vi "VIPMUninstallVIPackagesByName.vi"   [LabVIEW 2016]
uses:
  <vilib>/Wiresmith Technology/G CLI/Argument Parser/Option Class/Option Configuration.ctl
  <vilib>/Wiresmith Technology/G CLI/Argument Parser/Option Class/Argument Type.ctl
  <vilib>/Wiresmith Technology/G CLI/CLI Class/CLI.lvclass
  <vilib>/Wiresmith Technology/G CLI/Argument Parser/Option Set Class/Option Set.lvclass
  <vilib>/Wiresmith Technology/G CLI/Argument Parser/Option Class/Option.lvclass
  <vilib>/JKI/VIPM API/VIPM API_vipm_api.lvlib
types:
  T1 = typedef "Option Parser.lvlib/Option.lvclass/Option Configuration.ctl" = cluster{"Option Type":T2, "Option Labels":string[], "Key":string, "Description":string, "Required":bool, "Default Value":string}
  T2 = typedef "Option Parser.lvlib/Option.lvclass/Argument Type.ctl" = enum16{"flag", "value"}
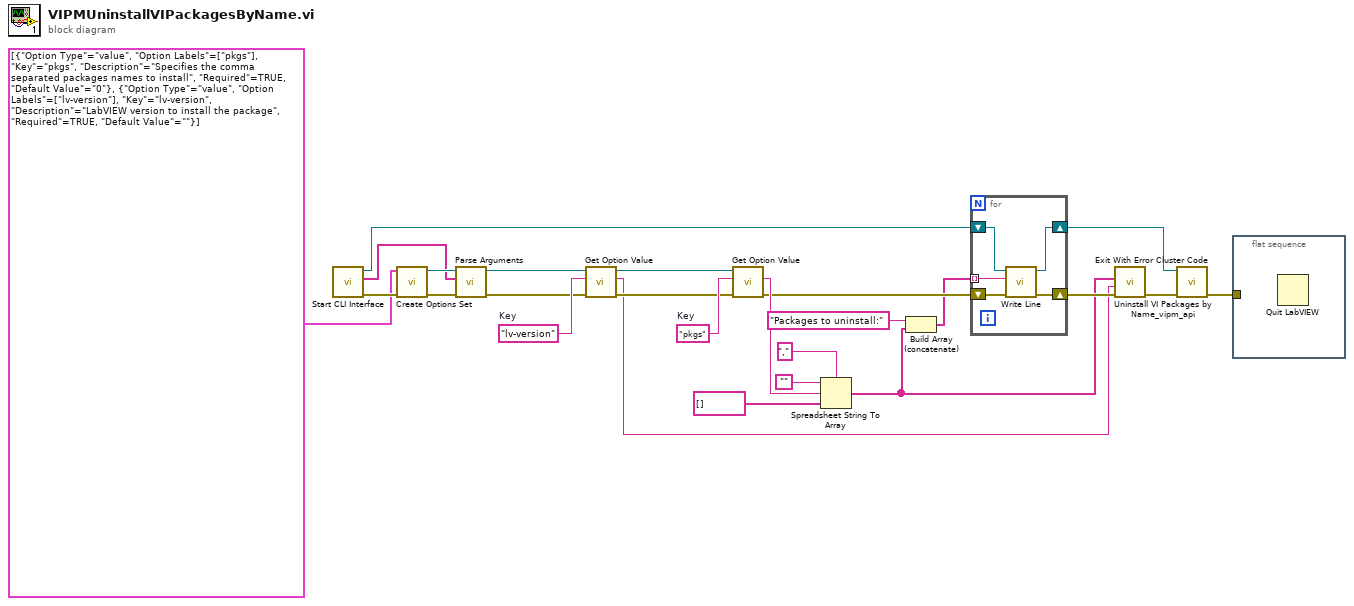
[diagram p0: block diagram]
diagram:
  w12 = "lv-version"  # Key
  w19 = "pkgs"  # Key
  n1 = call <vilib>:"Start CLI Interface.vi"() -> ("error out"=w21:errorcluster, "Custom Parameters"=w22:string[], "CLI out"=w25:refnum<class "CLI.lvclass">)  [unwired: 8 in, 1 out]
  n2 = call <vilib>:"Create Options Set.vi"("error in (no error)"=w21, "Options"=T1[] [{"Option Type"=enum."value", "Option Labels"=["pkgs"], "Key"="pkgs", "Description"="Specifies the comma separated packages names to install", "Required"=TRUE, "Default Value"="0"}, {"Option Type"=enum."value", "Option Labels"=["lv-version"], "Key"="lv-version", "Description"="LabVIEW version to install the package", "Required"=TRUE, "Default Value"=""}]) -> ("error out"=w23:errorcluster, "Option Set out"=w24:refnum<class "Option Set.lvclass">)  [unwired: 8 in]
  n3 = call <vilib>:"Parse Arguments.vi"("error in (no error)"=w23, "Arguments"=w22, "Option Set in"=w24) -> ("error out"=w11:errorcluster, "Option Set out"=w8:refnum<class "Option Set.lvclass">)  [unwired: 5 in, 2 out]
  n4 = call <vilib>:"Get Option Value.vi"("error in (no error)"=w11, "Option Key"=w12, "Option Set in"=w8) -> ("error out"=w10:errorcluster, "Value"=w7:string, "Option Set out"=w9:refnum<class "Option Set.lvclass">)  [unwired: 5 in, 1 out]
  n5 = call <vilib>:"Get Option Value.vi"("error in (no error)"=w10, "Option Key"=w19, "Option Set in"=w9) -> ("error out"=w4:errorcluster, "Value"=w6:string)  [unwired: 5 in, 2 out]
  n6 = Spreadsheet String To Array(delimiter (Tab)=",", format string="", spreadsheet string=w6, array type (2D Dbl)=string[] [] ("Value")) -> (array=w2:string[])
  n7 = Build Array (concatenate)("Packages to uninstall:" ("delimiter (Tab)"), w2) -> (w1:string[])
  n8 = for {
    shift-right: [w28] -> w15
    shift-left: w25 -> [w30]
    shift-right: [w29] -> w17
    shift-left: w4 -> [w27]
    tunnel: w1 -> [w26] mode=indexing
    n9 = call <vilib>:"Write Line.vi"("error in (no error)"=w27, "Text to Write"=w26, "CLI in"=w30) -> ("error out"=w29:errorcluster, "CLI out"=w28:refnum<class "CLI.lvclass">)  [unwired: 7 in]
  }
  n10 = call <vilib>:"Uninstall VI Packages by Name_vipm_api.vi"("error in (no error)"=w17, "LabVIEW Version"=w7, "Package Names to Uninstall []"=w2) -> ("error out"=w16:errorcluster)  [unwired: 8 in]
  n11 = call <vilib>:"Exit With Error Cluster Code.vi"("error in (no error)"=w16, "CLI in"=w15) -> ("error out"=w18:errorcluster)  [unwired: 9 in]
  n12 = flat-sequence {
    tunnel: w18 -> [_]
    frame #0 {
      n13 = Quit LabVIEW() -> ()  [unwired: 1 in]
    }
  }
